vi "SrvErrorText.vi"(1 "ErrNo":i32) -> (0 "ErrMessage":string)   [LabVIEW 2020, in "Snap7.lvlib"]
uses:
  Snap7.lvlib
  windows/lv_snap7.dll
panel:
  out "Error":bool
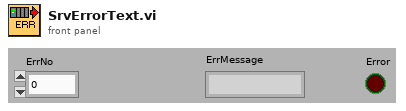
[diagram p1: front panel]
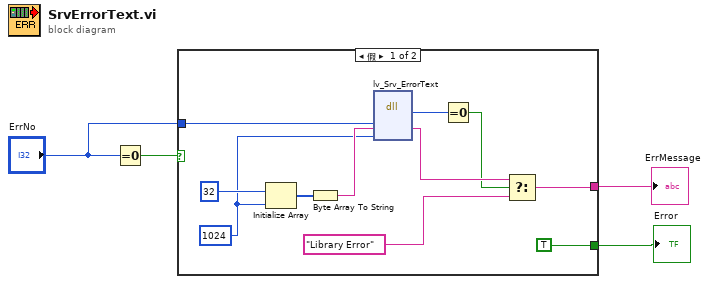
[diagram p0: block diagram]
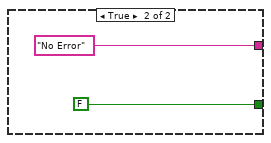
[diagram p2: hidden frame]
diagram:
  n1 = Equal To 0?(x="ErrNo") -> (x = 0?=w4:bool)
  n2 = case shown="假" w4 {
    tunnel: [w11 "No Error" ("f")] -> w3
    tunnel: "ErrNo" -> [w15 _]
    tunnel: [TRUE FALSE] -> w1
    frame False {
      w6 = 1024 ("Dimension Size")
      n3 = Initialize Array(u8 32 ("Element Data"), w6) -> (w14:u8[])
      n4 = Byte Array To String(unsigned byte array=w14) -> (string=w12:string)
      n5 = dll-call lib="PTH2fabs CUsersFeng项目HLCEPS300-2性能试验台SourcesSnap7libwindowslv_snap7.dll" fn="lv_Srv_ErrorText"("Error"=w15, "ErrMessage"=w12, "TextLen"=w6) -> ("return type"=w8:i32, "ErrMessage"=w10:string)  [unwired: 5 in, 2 out]
      n6 = Equal To 0?(x=w8) -> (x = 0?=w7:bool)
      n7 = Select(t=w10, s=w7, f="Library Error") -> (s? t:f=w11:string)
    }
    frame True {
    }
  }
  "ErrMessage" <- w3
  "Error" <- w1
